vi "Movie_read.vi"() -> ()   [LabVIEW 2025]
panel:
  in  "Path":path=path "/Users/crogers/Desktop/IMG_2932.mov"
  in  "Zoom Factor":sgl(slide) scale=0.0..1.0
  out "new picture":picture
  out "return value":u8[][][](array[numeric])
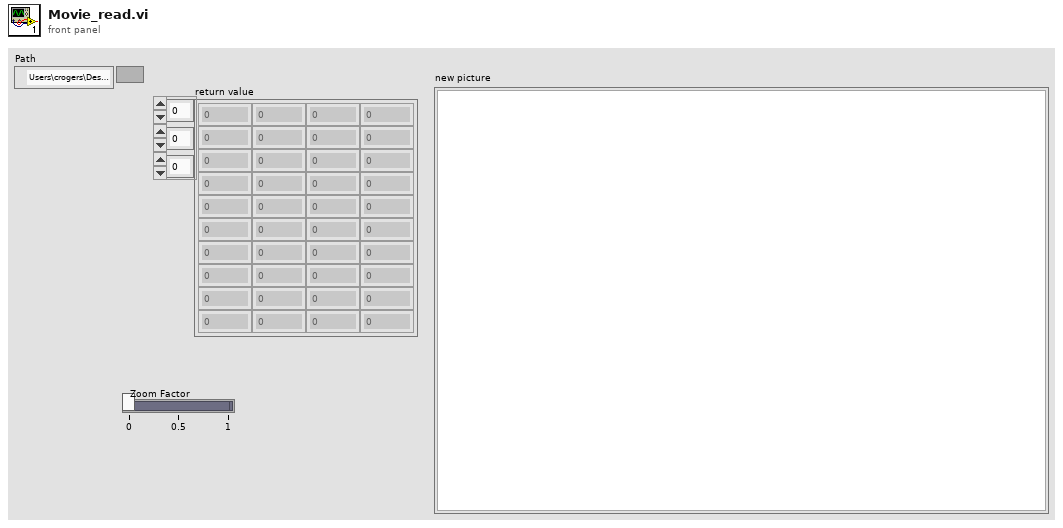
[diagram p1: front panel]
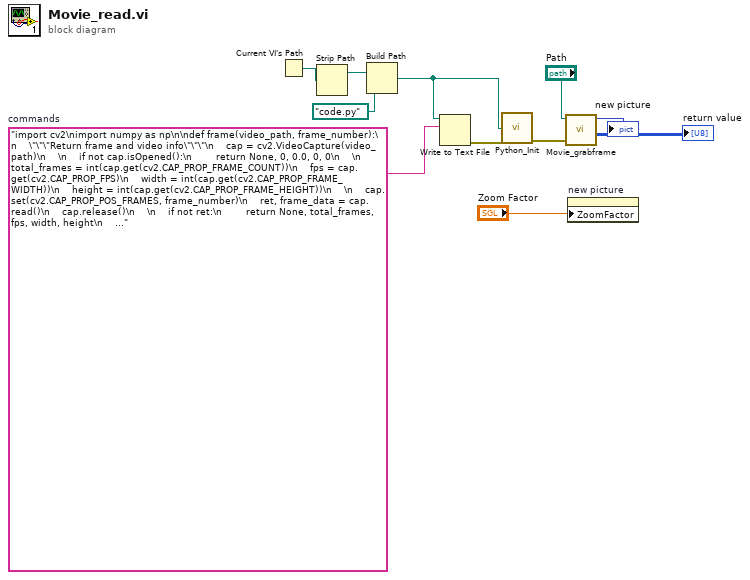
[diagram p0: block diagram]
diagram:
  w8 = "import cv2\nimport numpy as np\n\ndef frame(video_path, frame_number):\n    \"\"\"Return frame and video info\"\"\"\n    cap = cv2.VideoCapture(video_path)\n    \n    if not cap.isOpened():\n        return None, 0, 0.0, 0, 0\n    \n    total_frames = int(cap.get(cv2.CAP_PROP_FRAME_COUNT))\n    fps = cap.get(cv2.CAP_PROP_FPS)\n    width = int(cap.get(cv2.CAP_PROP_FRAME_WIDTH))\n    height = int(cap.get(cv2.CAP_PROP_FRAME_HEIGHT))\n    \n    cap.set(cv2.CAP_PROP_POS_FRAMES, frame_number)\n    ret, frame_data = cap.read()\n    cap.release()\n    \n    if not ret:\n        return None, total_frames, fps, width, height\n    \n    frame_rgb = cv2.cvtColor(frame_data, cv2.COLOR_BGR2RGB)\n    \n    return frame_rgb, total_frames, fps, width, height"  # commands
  n1 = Current VI's Path() -> (path=w10:path)
  n2 = Strip Path(path=w10) -> (stripped path=w9:path)  [unwired: 1 out]
  n3 = Build Path(base path=w9, name or relative path=path "code.py" ("file (use dialog)")) -> (appended path=w2:path)
  n4 = Write to Text File(file (use dialog)=w2, text=w8) -> (error out=w4:errorcluster)  [unwired: 2 in, 2 out]
  n5 = call "Python_Init.vi"("code in"=w2, "error in (no error)"=w4) -> ("error out"=w3:errorcluster)  [unwired: 2 in, 2 out]
  n6 = call "Movie_grabframe.vi"("error in (no error)"=w3, "Path"="Path") -> ("return value"=→"return value":u8[][][], "new picture"=→"new picture":picture)  [unwired: 6 in, 2 out]
  n7 = property on="new picture" class="Pict"("ZoomFactor"="Zoom Factor") -> ()  [unwired: 2 in, 2 out]
